vi "Write Raw.vi"(8 "error in (no error)":errorcluster, 10 "Data":u8[](array[numeric]), 11 "senseHatDisplay in":refnum<class "RPI.SenseHat.Display.lvclass">) -> (0 "error out":errorcluster, 3 "senseHatDisplay out":refnum<class "RPI.SenseHat.Display.lvclass">)   [LabVIEW 2020, in "RPI.SenseHat.Display.lvlib" / "RPI.SenseHat.Display.lvclass"]
doc: "Writes raw data to the physical display. The raw buffer must be 192 bytes long.\nThe layout of the LED buffer:\n Row 1: R R R R R R R R G G G G G G G G B B B B B B B B\n Row 2: R R R R R R R R G G G G G G G G B B B B B B B B\n ...\n Row 8: R R R R R R R R G G G G G G G G B B B B B B B B\n\nNote: Each color component is only 5 bits long, i.e. 0=darkest and 31=brightest."
uses:
  RPI.SenseHat.Display.lvclass
  RPI/Classes/mainI2CDevice/mainI2CDevice.lvclass
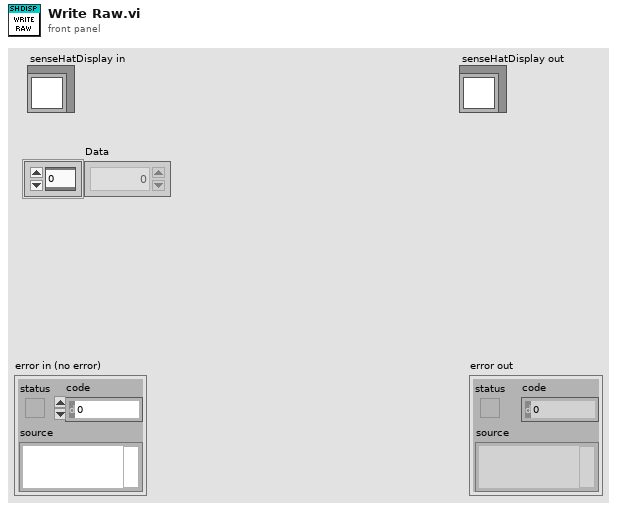
[diagram p1: front panel]
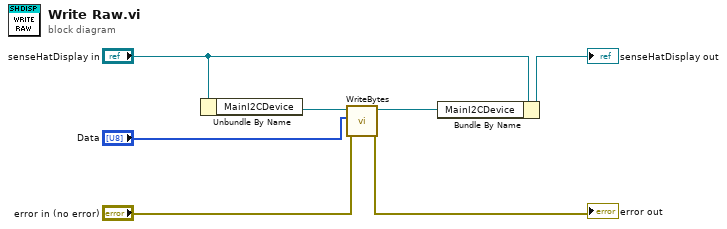
[diagram p0: block diagram]
diagram:
  n1 = Unbundle By Name("senseHatDisplay in") -> ("MainI2CDevice"=w5:refnum<class "mainI2CDevice.lvclass">)
  n2 = call "WriteBytes.vi"("error in (no error)"="error in (no error)", "Data"="Data", "mainI2CDevice in"=w5) -> ("error out"=→"error out":errorcluster, "mainI2CDevice out"=w4:refnum<class "mainI2CDevice.lvclass">)  [unwired: 7 in]
  n3 = Bundle By Name(cluster="senseHatDisplay in", "MainI2CDevice"=w4) -> (→"senseHatDisplay out":refnum<class "RPI.SenseHat.Display.lvclass">)
